vi "VectorNav Read Data.vi"() -> ()   [LabVIEW 2009]
uses:
  VectorNav DFA States.ctl
panel:
  in  "VectorNav Raw Data":u8
  out "Boolean":bool
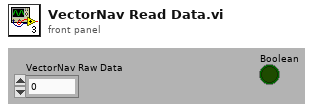
[diagram p1: front panel]
types:
  T1 = typedef "VectorNav DFA States.ctl" = enum16{"confirm check sum", "check status byte", "read measured values", "confirm measurement", "confirm command", "read message length", "read address", "wait for \"02\""}
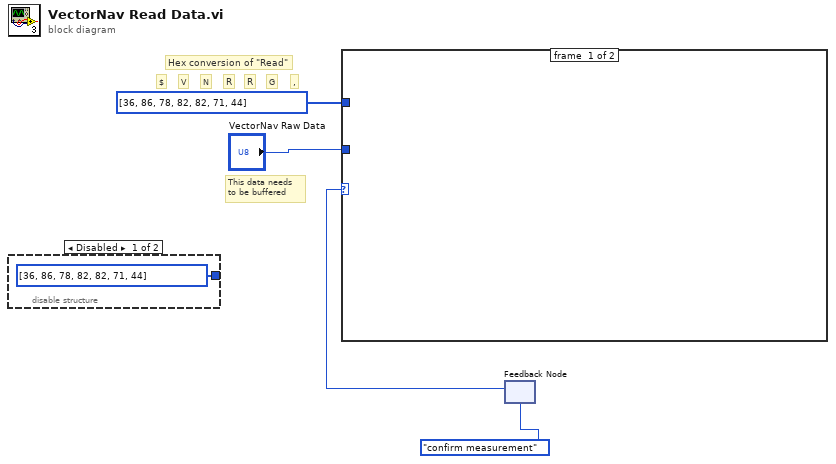
[diagram p0: block diagram]
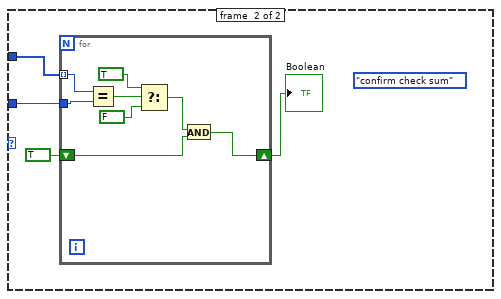
[diagram p2: hidden frame]
diagram:
  # "This data needs\nto be buffered"
  # "Hex conversion of \"Read\""
  # ","
  # "G"
  # "R"
  # "R"
  # "N"
  # "V"
  # "$"
  n1 = disable-structure shown="Disabled" {
    disable-tunnel: [u8[] [36, 86, 78, 82, 82, 71, 44] _] -> _
    frame #0 {
    }
    frame #1 {
    }
  }
  n2 = feedback #1(VectorNav_DFA_States."confirm measurement" ("Enum")) -> (w1:T1)
  n3 = case shown="\"check status byte\"" w1 {
    tunnel: u8[] [36, 86, 78, 82, 82, 71, 44] -> [_ w9]
    tunnel: "VectorNav Raw Data" -> [_ w6]
    frame #0 {
    }
    frame #1 {
      (unwired) VectorNav_DFA_States."confirm check sum" ("Enum")
      n4 = for {
        tunnel: w9 -> [w17] mode=indexing
        tunnel: w6 -> [w16]
        shift-right: [w11] -> w7
        shift-left: TRUE -> [w10]
        n5 = Equal?(x=w17, y=w16) -> (x = y?=w15:bool)
        n6 = Select(t=TRUE, s=w15, f=FALSE) -> (s? t:f=w12:bool)
        n7 = And(x=w12, y=w10) -> (x .and. y?=w11:bool)
      }
      "Boolean" <- w7
    }
  }
